vi "Actor Core.vi"(8 "error in":errorcluster, 11 "BasicTerminalBinding In":refnum<class "BasicTerminalBinding.lvclass">) -> (0 "error out":errorcluster, 3 "Actor out":refnum<class "Actor.lvclass">)   [LabVIEW 2020, in "TestViewables.lvlib" / "BasicTerminalBinding.lvclass"]
doc: "(<B>Filename</B>: Actor Framework.lvlib:Actor.lvclass:Actor Core.vi)\n\nReceives messages to the actor, reacts to them, and initiates any error handling that may shut the actor down.\n\nDescendant classes may override this VI to append parallel tasks for the actor to complete while it handles messages. Overrides use the Call Parent Method node.\n\n<License>\nCopyright © 2017 Composed Systems, LLC | All rights reserved\nwww.composed.io\n\nAuthor: Ethan Stern <ethan.stern@composed.io>\n\nThis software is provided \"AS IS\" WITHOUT WARRANTIES, either express or implied, AND IS FOR EDUCATIONAL PURPOSES ONLY.\n</License>"
uses:
  BasicTerminalBinding.lvclass
  C:/Program Files/National Instruments/LabVIEW 2020/vi.lib/ActorFramework/Actor/Actor.lvclass
  <vilib>/ActorFramework/Actor/Actor.lvclass
  BasicTerminalBinding.lvclass/BasicTerminalBinding.ctl
  <vilib>/ActorFramework/Actor/Actor.lvclass/Actor.ctl
  <vilib>/ActorFramework/Message Enqueuer/Message Enqueuer.lvclass/Message Enqueuer.ctl
  modules/mva-core/Source/SubscriptionPolicy/ValueChangeSubscription/ValueChangeSubscription.lvclass/ValueChangeSubscription.ctl
  modules/mva-core/Source/IObserver/IObserver Messages/Observe Data Msg/Observe Data Msg.lvclass/Observe Data Msg.ctl
  modules/composed-af-messages/Source/RoundTripMessage/RoundTripMessage.lvclass/RoundTripMessage.ctl
  modules/mva-core/Source/IObserver/ActorDataBinding/ActorDataBinding.lvclass/ActorDataBinding.ctl
  modules/mva-core/Source/IMediator/SubscriptionRequest/SubscriptionRequest.lvclass/SubscriptionRequest.ctl
  modules/mva-core/Source/IObserver/IObserver Messages/Subscribe Msg/Subscribe Msg.lvclass/Subscribe Msg.ctl
  962bf76c-2fa4-4b61-b2f2-59132d242665.vi
  modules/mva-core/Source/IMediator/SubscriptionRequest/Pack Subscription Request.vi
  modules/mva-core/Source/SubscriptionPolicy/BasicSubscription/New Basic Subscription.vi
  modules/mva-core/Source/SubscriptionPolicy/ValueChangeSubscription/New Value Change Subscription.vi
  modules/mva-core/Source/IObserver/ActorDataBinding/New Actor Data Binding Transport.vi
  modules/mva-core/Source/IObserver/IObserver Messages/Subscribe Msg/Send Subscribe.vi
  <vilib>/ActorFramework/Actor/Read Self Enqueuer.vi
  modules/mva-core/Source/IObserver/IObserver Messages/Observe Data Msg/Write Observe Data Msg Return Info.vi
  <vilib>/ActorFramework/Message Enqueuer/Enqueue.vi
  <vilib>/ActorFramework/Message Enqueuer/Init from Existing Queue.vi
  modules/composed-af-messages/Source/RoundTripMessage/Write Return Address.vi
  modules/mva-core/Source/SubscriptionPolicy/ValueChangeSubscription/ValueChangeSubscription.lvclass
  modules/mva-core/Source/IObserver/IObserver Messages/Observe Data Msg/Observe Data Msg.lvclass
  modules/mva-core/Source/IObserver/ActorDataBinding/ActorDataBinding.lvclass
  modules/mva-core/Source/IObserver/IObserver Messages/Subscribe Msg/Subscribe Msg.lvclass
  C:/Program Files/National Instruments/LabVIEW 2020/vi.lib/ActorFramework/Message/Message.lvclass
  modules/mva-core/Source/IMediator/ISubscriptionPolicy/Open Subscription Policy.vi
  <vilib>/Utility/error.llb/Error Cluster From Error Code.vi
  <vilib>/ActorFramework/Message Priority Queue/Priority Enqueue.vi
  modules/mva-core/Source/SubscriptionPolicy/BasicSubscription/BasicSubscription.lvclass
  <vilib>/ActorFramework/Message Enqueuer/Message Enqueuer.lvclass
  modules/mva-core/Source/IMediator/SubscriptionRequest/SubscriptionRequest.lvclass
  modules/mva-viewable/Source/IViewable/IViewable/IViewable.lvclass
panel:
  out "Random Number":dbl format="%.3f"
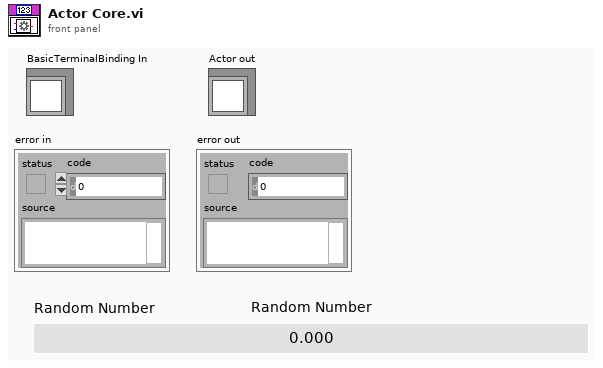
[diagram p1: front panel]
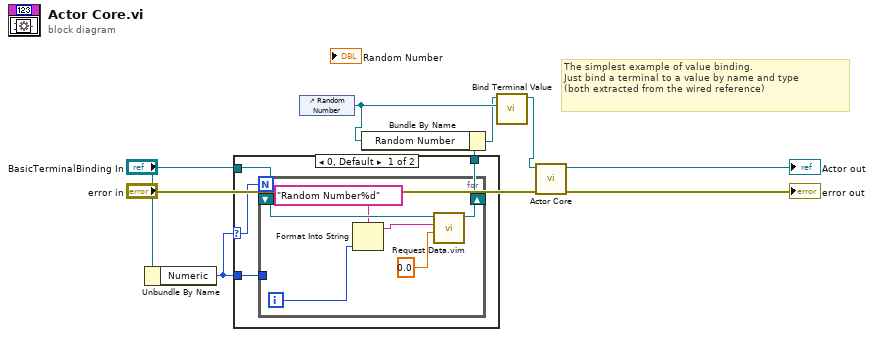
[diagram p0: block diagram]
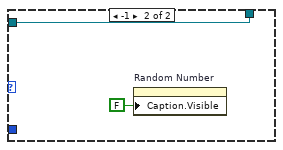
[diagram p2: hidden frame]
diagram:
  # "The simplest example of value binding.\nJust bind a terminal to a value by name and type\n(both extracted from the wired reference)"
  n1 = Unbundle By Name("BasicTerminalBinding In") -> ("Numeric"=w1:i32)
  n2 = case shown="0, Default" w1 {
    selector: w1 -> [w10 _]
    tunnel: [w13 w21] -> w5
    tunnel: "BasicTerminalBinding In" -> [w12 w21]
    tunnel: w1 -> [w11 _]
    frame 0, Default {
      n3 = for {
        N: w10 -> [_]
        tunnel: w11 -> [_]
        shift-right: [w19] -> w13
        shift-left: w12 -> [w18]
        i -> [w14]
        n4 = Format Into String(format string="Random Number%d", w14) -> (resulting string=w16:string)  [unwired: 2 in, 1 out]
        n5 = call "Request Data.vim"("Data Type"=0.0 ("Random Number"), "Datum Name"=w16, "IObserver in"=w18) -> ("IObserver out"=w19:refnum<class "BasicTerminalBinding.lvclass">)  [unwired: 6 in, 2 out]
      }
    }
    frame -1 {
      n6 = property on="Random Number" class="DigNum (strict)"("Caption.Visible"=FALSE) -> ()  [unwired: 2 in, 2 out]
    }
  }
  n7 = control-ref of="Random Number"() -> (w6:refnum<vi>)
  n8 = Bundle By Name(cluster=w5, "Random Number"=w6) -> (w4:refnum<class "BasicTerminalBinding.lvclass">)
  n9 = call "Bind Terminal Value.vi"("Ctl Refnum"=w6, "IViewable in"=w4) -> ("IViewable out"=w3:refnum<class "BasicTerminalBinding.lvclass">)  [unwired: 8 in, 1 out]
  n10 = call-parent "Actor Core.vi"("error in"="error in", "IViewable In"=w3) -> ("error out"=→"error out":errorcluster, "Actor out"=→"Actor out":refnum<class "Actor.lvclass">)  [unwired: 8 in]
